vi "Block Tree UI.vi"() -> ()   [LabVIEW 2022 SP3, in "FlexBlocks Support.lvlib"]
uses:
  FlexBlocks Support.lvlib
panel:
  in  "Block Tree":string(tree)
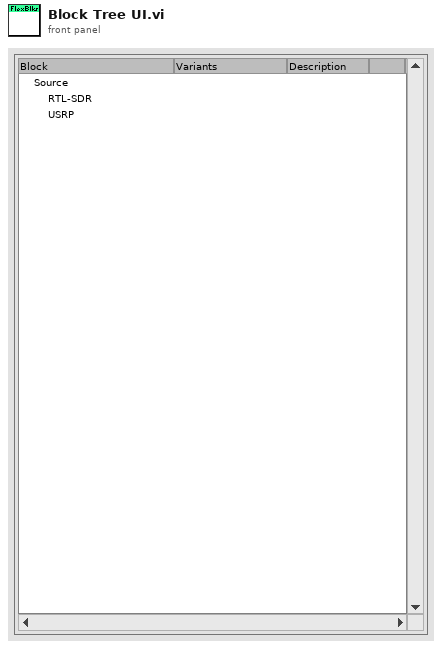
[diagram p1: front panel]
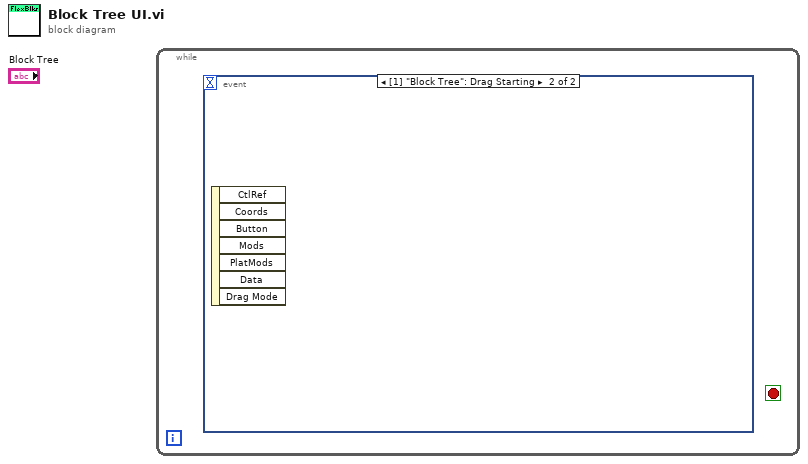
[diagram p0: block diagram]
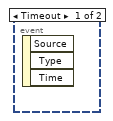
[diagram p2: hidden frame]
diagram:
  n1 = while {
    stop <- _ stop-if-true
    n2 = event shown="[1] \"Block Tree\": Drag Starting" {
      selector: _ -> [_ _]
      dyn-events: _ -> [_ _]
      timeout: _ -> [_ _]
      event Timeout {
        n3 = event-data() -> ()  [unwired: 1 in, 3 out]
      }
      event "Block Tree": Drag Starting {
        n4 = event-data() -> ()  [unwired: 1 in, 7 out]
      }
    }
  }
